vi "Set gRPC ID.vi"(10 "gRPC ID":T1, 11 "OOP Server in":refnum<class "Ex1_server.lvclass">) -> (3 "OOP Server out":refnum<class "Ex1_server.lvclass">)   [LabVIEW 2019, in "Ex1_server.lvlib" / "Ex1_server.lvclass"]
uses:
  Ex1_server.lvclass
  <vilib>/gRPC/LabVIEW gRPC Library/Server API/typeDefs/grpcId.ctl
  Ex1_server.lvclass/Ex1_server.ctl
  <vilib>/gRPC/LabVIEW gRPC Library/gprc-lvsupport-release.lvlib
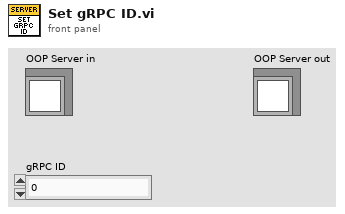
[diagram p1: front panel]
types:
  T1 = typedef "gprc-lvsupport-release.lvlib/grpcId.ctl" = u64
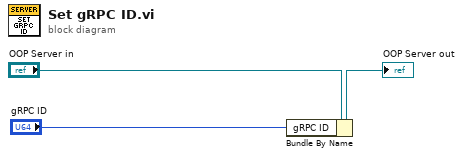
[diagram p0: block diagram]
diagram:
  n1 = Bundle By Name(cluster="OOP Server in", "gRPC ID"="gRPC ID") -> (→"OOP Server out":refnum<class "Ex1_server.lvclass">)
